vi "Write Value (variant).vi"(8 "error in (no error)":errorcluster, 10 "Variant":variant, 11 "Floating point base in":refnum<class "Floating point base.lvclass">) -> (0 "error out":errorcluster, 3 "Floating point base out":refnum<class "Floating point base.lvclass">)   [LabVIEW 2018, in "D Datagrid Library.lvlib" / "Floating point base.lvclass"]
uses:
  Floating point base.lvclass
  DatagridElement/DatagridElement.lvclass
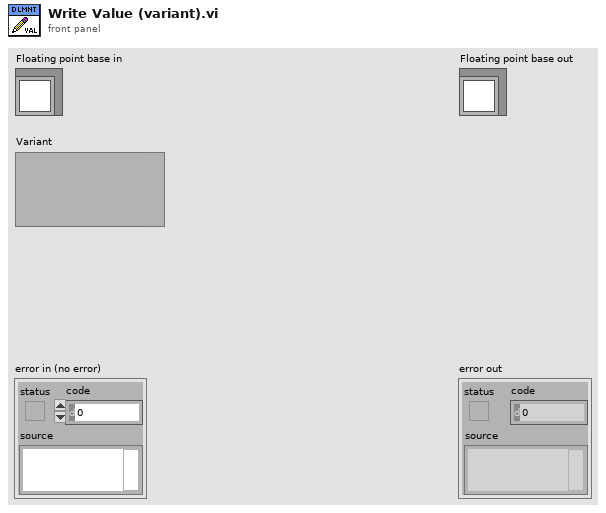
[diagram p1: front panel]
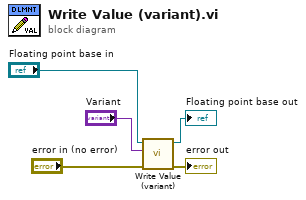
[diagram p0: block diagram]
diagram:
  n1 = call-parent "Write Value (variant).vi"("error in (no error)"="error in (no error)", "Variant"="Variant", "DatagridElement in"="Floating point base in") -> ("error out"=→"error out":errorcluster, "DatagridElement out"=→"Floating point base out":refnum<class "Floating point base.lvclass">)  [unwired: 7 in]
